vi "GMLAN ClearDiagnosticInformation.vi"(8 "error in (no error)":errorcluster, 11 "diag ref in":T1) -> (0 "error out":errorcluster, 1 "success?":bool, 3 "diag ref out":T1)   [LabVIEW 2013, in "GMLAN.lvlib"]
uses:
  GMLAN.lvlib
  <vilib>/Automotive Diagnostic Command Set/Diagnostic Transport.llb/Diag Reference.ctl
  <vilib>/Automotive Diagnostic Command Set/Diagnostic Transport.llb/Transport Protocol Selector.ctl
  <vilib>/Automotive Diagnostic Command Set/Diagnostic Transport.llb/Diag CAN Frame Log.ctl
  <vilib>/Automotive Diagnostic Command Set/Diagnostic Transport.llb/Apply Diagnostic Error.vi
  <vilib>/Automotive Diagnostic Command Set/Diagnostic Transport.llb/Diag Globals.vi
  <vilib>/Automotive Diagnostic Command Set/Diagnostic Transport.llb/Diagnostic Service Send.vi
  <vilib>/Automotive Diagnostic Command Set/Diagnostic Transport.llb/Diagnostic Response Recv.vi
  <vilib>/addons/Automotive Diagnostic Command Set/NI_Automotive Diagnostic Command Set.lvlib
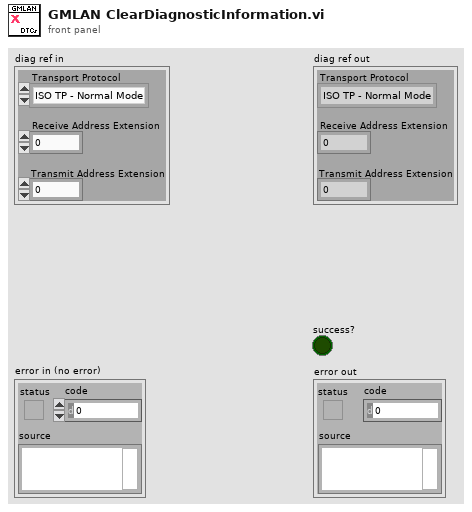
[diagram p1: front panel]
types:
  T1 = typedef "NI_Automotive Diagnostic Command Set.lvlib/Diag Reference.ctl" = cluster{"Diag CAN Handle":u32, "Transport Protocol":T2, "Receive Address Extension":u8, "Transmit Address Extension":u8, "Receive CAN Id":u32, "Transmit CAN Id":u32, "Diag CAN Queue":refnum<queue>, "Log Frames ?":bool, "My TP Address":u8, "Other TP Address":u8, "T1":u16, "T2":u16, "T3":u16, "T4":u16, "Tx SN":u8, "Block Size":u8, "Rx SN":u8, "VW TP Initialized?":bool, "Tx block no":u8, "baud rate":u32, "Interface":string, "Channel Diag CAN Handle":u32, "UDP Connection ID":refnum<k16>, "TCP Connection ID":refnum<k5>, "Target IP Addr":u32, "Source Address":u16, "Target Address":u16, "Send Header NACK?":bool, "DLL Handle":u32, "NAD":u8, "Time Stamp read first":dbl, "Time Stamp read last":dbl, "Time Stamp write first":dbl, "Time Stamp write last":dbl, "Time Stamp write":dbl, "Time Stamp read":dbl}
  T2 = typedef "NI_Automotive Diagnostic Command Set.lvlib/Transport Protocol Selector.ctl" = enum16{"ISO TP - Normal Mode", "ISO TP - Mixed Mode", "VW TP 2.0", "Diagnostics on IP", "ISO TP LIN"}
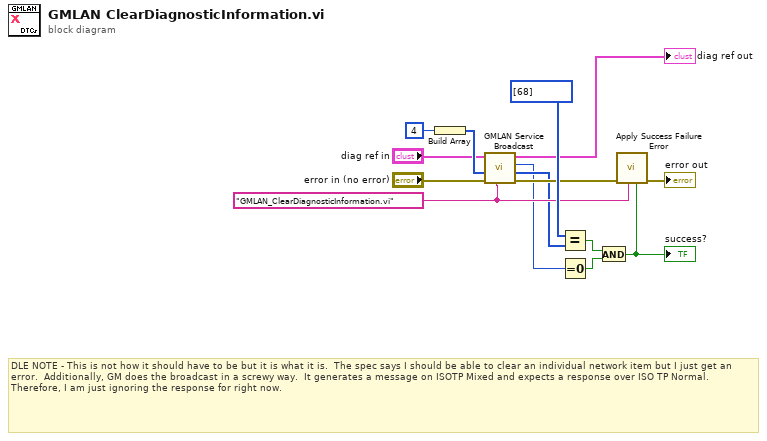
[diagram p0: block diagram]
diagram:
  w8 = "GMLAN_ClearDiagnosticInformation.vi" ("error source")
  # "DLE NOTE - This is not how it should have to be but it is what it is.  The spec says I should be able to clear an individual network item but I just get an error.  Additionally, GM does the broadcast in a screwy way.  It generates a message on ISOTP Mixed and expects a response over ISO TP Normal.  Therefore, I am just ignoring the response for right now."
  n1 = Build Array(u8 4 ("element")) -> (w9:u8[])
  n2 = call "GMLAN Service Broadcast.vi"("error source"=w8, "error in (no error)"="error in (no error)", "data in"=w9, "diag ref in"="diag ref in") -> ("error out"=w7:errorcluster, "data out"=w6:u8[], "error code"=w5:u8, "diag ref out"=→"diag ref out":T1)  [unwired: 4 in]
  n3 = Equal?(x=u8[] [68], y=w6) -> (x = y?=w2:bool)
  n4 = Equal To 0?(x=w5) -> (x = 0?=w1:bool)
  n5 = And(x=w2, y=w1) -> (x .and. y?=w11:bool)
  "success?" <- w11
  n6 = call <vilib>:"Apply Success Failure Error.vi"("success code"=w11, "error source"=w8, "error in (no error)"=w7) -> ("error out"=→"error out":errorcluster)  [unwired: 8 out]
